vi "error_detection_demoinfocom.vi"(9 "SDR2 Key before ECC":u8[](array[numeric]), 10 "SDR1 Key before ECC":u8[](array[numeric]), 11 "Quantization rate":dbl) -> (3 "Array":bool[][](array[boolean]))   [LabVIEW 2021]
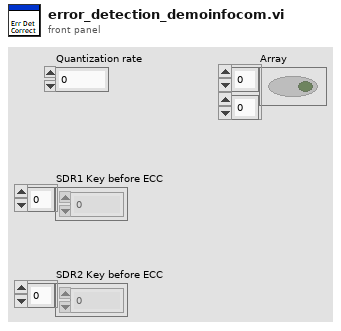
[diagram p1: front panel]
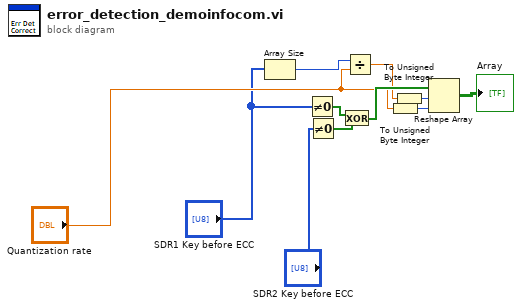
[diagram p0: block diagram]
diagram:
  n1 = Array Size(array="SDR1 Key before ECC") -> (size(s)=w6:i32)
  n2 = Not Equal To 0?(x="SDR1 Key before ECC") -> (x != 0?=w2:bool[])
  n3 = Not Equal To 0?(x="SDR2 Key before ECC") -> (x != 0?=w3:bool[])
  n4 = Exclusive Or(1:w3, 2:w2) -> (0:w10:bool[])
  n5 = Divide(x=w6, y="Quantization rate") -> (x/y=w9:dbl)
  n6 = To Unsigned Byte Integer(number="Quantization rate") -> (unsigned 8bit integer=w4:u8)
  n7 = To Unsigned Byte Integer(number=w9) -> (unsigned 8bit integer=w8:u8)
  n8 = Reshape Array(w10, w8, w4) -> (→"Array":bool[][])
